vi "GVmotor_Motor_enable.vi"(8 "error in (no error)":errorcluster, 11 "VISA resource name":refnum<visa-resource-name>) -> (0 "error out":errorcluster, 3 "VISA resource name out":refnum<visa-resource-name>)   [LabVIEW 2019]
panel:
  in  "milliseconds to wait":u32=100
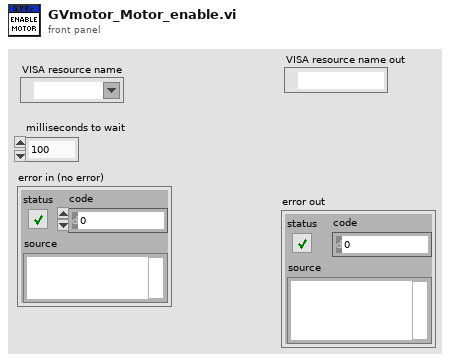
[diagram p1: front panel]
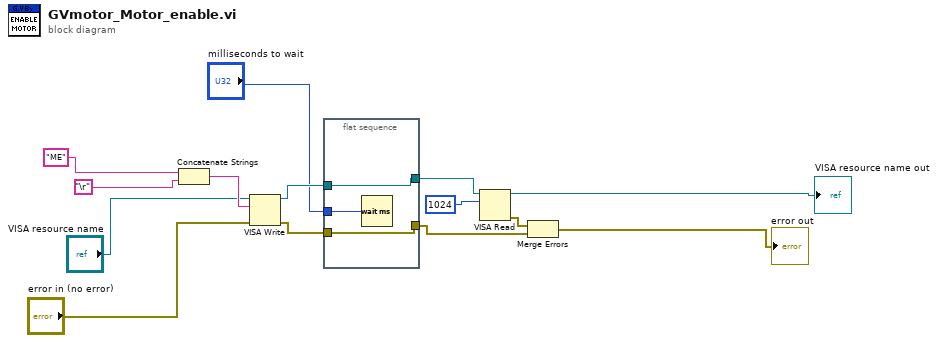
[diagram p0: block diagram]
diagram:
  n1 = Concatenate Strings("ME" ("string"), "\r") -> (w14:string)
  n2 = VISA Write(VISA resource name="VISA resource name", write buffer=w14, error in (no error)="error in (no error)") -> (VISA resource name out=w10:refnum<visa-resource-name>, error out=w11:errorcluster)  [unwired: 1 out]
  n3 = flat-sequence {
    tunnel: [w17] -> w6
    tunnel: w11 -> [w17]
    tunnel: [w16] -> w9
    tunnel: w10 -> [w16]
    tunnel: "milliseconds to wait" -> [w15]
    frame #0 {
      n4 = Wait (ms)(milliseconds to wait=w15) -> ()  [unwired: 1 out]
    }
  }
  n5 = VISA Read(VISA resource name=w9, byte count=u32 1024) -> (VISA resource name out=→"VISA resource name out":refnum<visa-resource-name>, error out=w5:errorcluster)  [unwired: 1 in, 2 out]
  n6 = Merge Errors(w5, w6) -> (→"error out":errorcluster)
